vi "concatenate name.vi"() -> ()   [LabVIEW 2020]
panel:
  out "full name":string
  in  "last name":string
  in  "first name":string
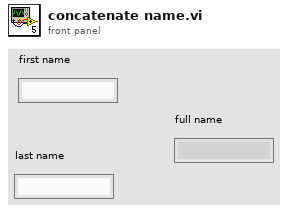
[diagram p1: front panel]
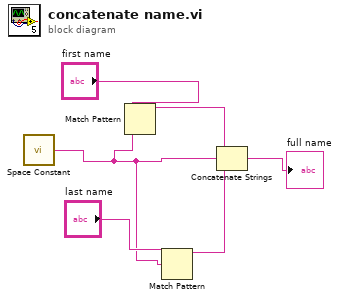
[diagram p0: block diagram]
diagram:
  n1 = call <vilib>:"Space Constant.vi"() -> ("String"=w1:string)
  n2 = Match Pattern(string="first name", regular expression=w1) -> (before substring=w3:string)  [unwired: 1 in, 3 out]
  n3 = Match Pattern(string="last name", regular expression=w1) -> (before substring=w2:string)  [unwired: 1 in, 3 out]
  n4 = Concatenate Strings(w3, w1, w2) -> (→"full name":string)
